vi "Move_Omni_Wheels_Servo.vi"(10 "Spin or not to spin":bool, 11 "Oculus Data":T2={"head"={"orientation"={"roll"=1.6327005330047937, "pitch"=-89.08559793078238, "yaw"=-40.95061142092874}, "position"={"x"=1.207441, "y"=0.483058, "z"=-0.742013}}, "hands"={"left"={"position"={"x"=inf, "y"=inf, "z"=-inf}, "orientation"={"roll"=-51.475846117481964, "pitch"=106.93248840397386, "yaw"=69.74254276716579}}, "right"={"position"={"x"=inf, "y"=inf, "z"=-inf}, "orientation"={"roll"=49.02272731762935, "pitch"=105.46319543414037, "yaw"=-123.9602784132463}}}, "buttons"={"a"=FALSE, "b"=FALSE, "x"=FALSE, "y"=FALSE, "menu"=FALSE, "leftTrig"=1e-06, "rightTrig"=1e-06, "leftGrip"=1e-06, "rightGrip"=1e-06, "left_jstick"={"x"=-0.002561, "y"=0.007201, "button"=FALSE}, "right_jstick"={"x"=0.0, "y"=0.0, "button"=FALSE}}}) -> (3 "2D Picture":picture)   [LabVIEW 2017]
uses:
  <vilib>/myRIO/Instrument Drivers/Onboard IO/PWM/typedefs/PWM Reference.ctl
  <vilib>/myRIO/Common/Instrument Driver Framework/Utilities/typedefs/myRIO Generic Hardware Reference.ctl
  <vilib>/myRIO/Common/Instrument Driver Framework/Utilities/typedefs/Hardware Version Enum.ctl
  <vilib>/myRIO/Common/Instrument Driver Framework/Utilities/typedefs/myRIO v1.0 Reference.ctl
  <vilib>/myRIO/Common/Instrument Driver Framework/Utilities/typedefs/Generic FPGA Reference.ctl
  <vilib>/myRIO/Common/Instrument Driver Framework/myRIO v1.0/PWM/typedefs/PWM Channels Enum.ctl
  <vilib>/myRIO/Instrument Drivers/Onboard IO/PWM/typedefs/PWM Configuration.ctl
  <vilib>/userdefined/High Color/nirio_resource_hc.ctl
  <vilib>/myRIO/Common/Instrument Driver Framework/Utilities/vis/Is FPGA Ref Available.vi
  <vilib>/myRIO/Common/Instrument Driver Framework/myRIO v1.0/PWM/vis/myRIO v1.1 Open PWM.vi
  <vilib>/myRIO/Instrument Drivers/Onboard IO/PWM/vis/Set Duty Cycle and Frequency.vi
  <vilib>/myRIO/Common/Instrument Driver Framework/Utilities/vis/Validate Channels.vi
  <vilib>/myRIO/Common/Instrument Driver Framework/myRIO v1.0/PWM/vis/myRIO v1.0 Reserve PWM.vi
  <vilib>/myRIO/Common/Instrument Driver Framework/myRIO v1.0/PWM/vis/myRIO v1.0 Build MUX Configuration PWM.vi
  <vilib>/myRIO/Common/Instrument Driver Framework/myRIO v1.0/Resource Manager/vis/myRIO v1.0 Reserve Channel List.vi
  <vilib>/myRIO/Common/Instrument Driver Framework/myRIO v1.0/Resource Manager/vis/myRIO v1.0 Create Configuration List.vi
  <vilib>/myRIO/Common/Instrument Driver Framework/myRIO v1.0/Resource Manager/vis/myRIO v1.0 Reserve Channel.vi
  <vilib>/myRIO/Common/Instrument Driver Framework/myRIO v1.0/Resource Manager/vis/myRIO v1.0 Unreserve Channel.vi
  <vilib>/myRIO/Common/Instrument Driver Framework/myRIO v1.0/Resource Manager/vis/myRIO v1.0 Build Mutex Name.vi
  <vilib>/Utility/VariantDataType/GetNumericInfo.vi
  <vilib>/Utility/error.llb/Error Cluster From Error Code.vi
  <vilib>/myRIO/Common/Instrument Driver Framework/myRIO v1.0/myRIO v1.1 Open.vi
  <vilib>/myRIO/Common/Instrument Driver Framework/Utilities/vis/IO Manager.vi
  <vilib>/myRIO/Common/Instrument Driver Framework/Utilities/vis/Configuration Manager.vi
  <vilib>/myRIO/Common/Instrument Driver Framework/myRIO v1.0/Resource Manager/vis/myRIO v1.0 Configure IO.vi
  <vilib>/myRIO/Common/Instrument Driver Framework/myRIO v1.0/myRIO v1.0 Close.vi
  <vilib>/myRIO/Common/Instrument Driver Framework/myRIO v1.0/PWM/vis/myRIO v1.0 Write PWM.vi
  <vilib>/express/express arith-compare/Formula/XNode/ExpressFormulaBlockNode.xnode
  <vilib>/myRIO/Express VI/Onboard IO/PWM/PWM Express VI.xnode
  <vilib>/myRIO/Instrument Drivers/Onboard IO/PWM/vis/myRIO PWM Open.xnode
  <vilib>/myRIO/Instrument Drivers/Onboard IO/PWM/PWM.lvlib
panel:
  in  "rect":T1={"left"=0, "top"=0, "right"=407, "bottom"=407}
  out "r scaled":dbl=1e-06
  in  "Arrow Size":dbl=15.0 format="%#_13g"
  in  "Rotation Radius":dbl=50.0 format="%#_13g"
  out "SuMM":dbl(slide)=2.168404344971009e-18 scale=-3.0..3.0
  out "M3 Slider":dbl(slide)=-0.004955748932651739 scale=-1.0..1.0
  out "M2 Slider":dbl(slide)=0.007516748932651743 scale=-1.0..1.0
  out "M1 Slider":dbl(slide)=-0.002561000000000002 scale=-1.0..1.0
  out "Duty 3":dbl=0.075
  out "Duty 2":dbl=0.075
  out "Duty 1":dbl=0.075
  out "buttons.rightGrip":dbl=1e-06
  out "buttons.leftGrip":dbl=1e-06
  out "RightJoyStick X":dbl(slide) scale=-1.0..1.0
  out "X":dbl=-0.002561
  out "M 3":dbl=-0.004955748932651739
  out "M 2":dbl=0.007516748932651743
  out "M 1":dbl=-0.002561000000000002
  out "Y":dbl=0.007201
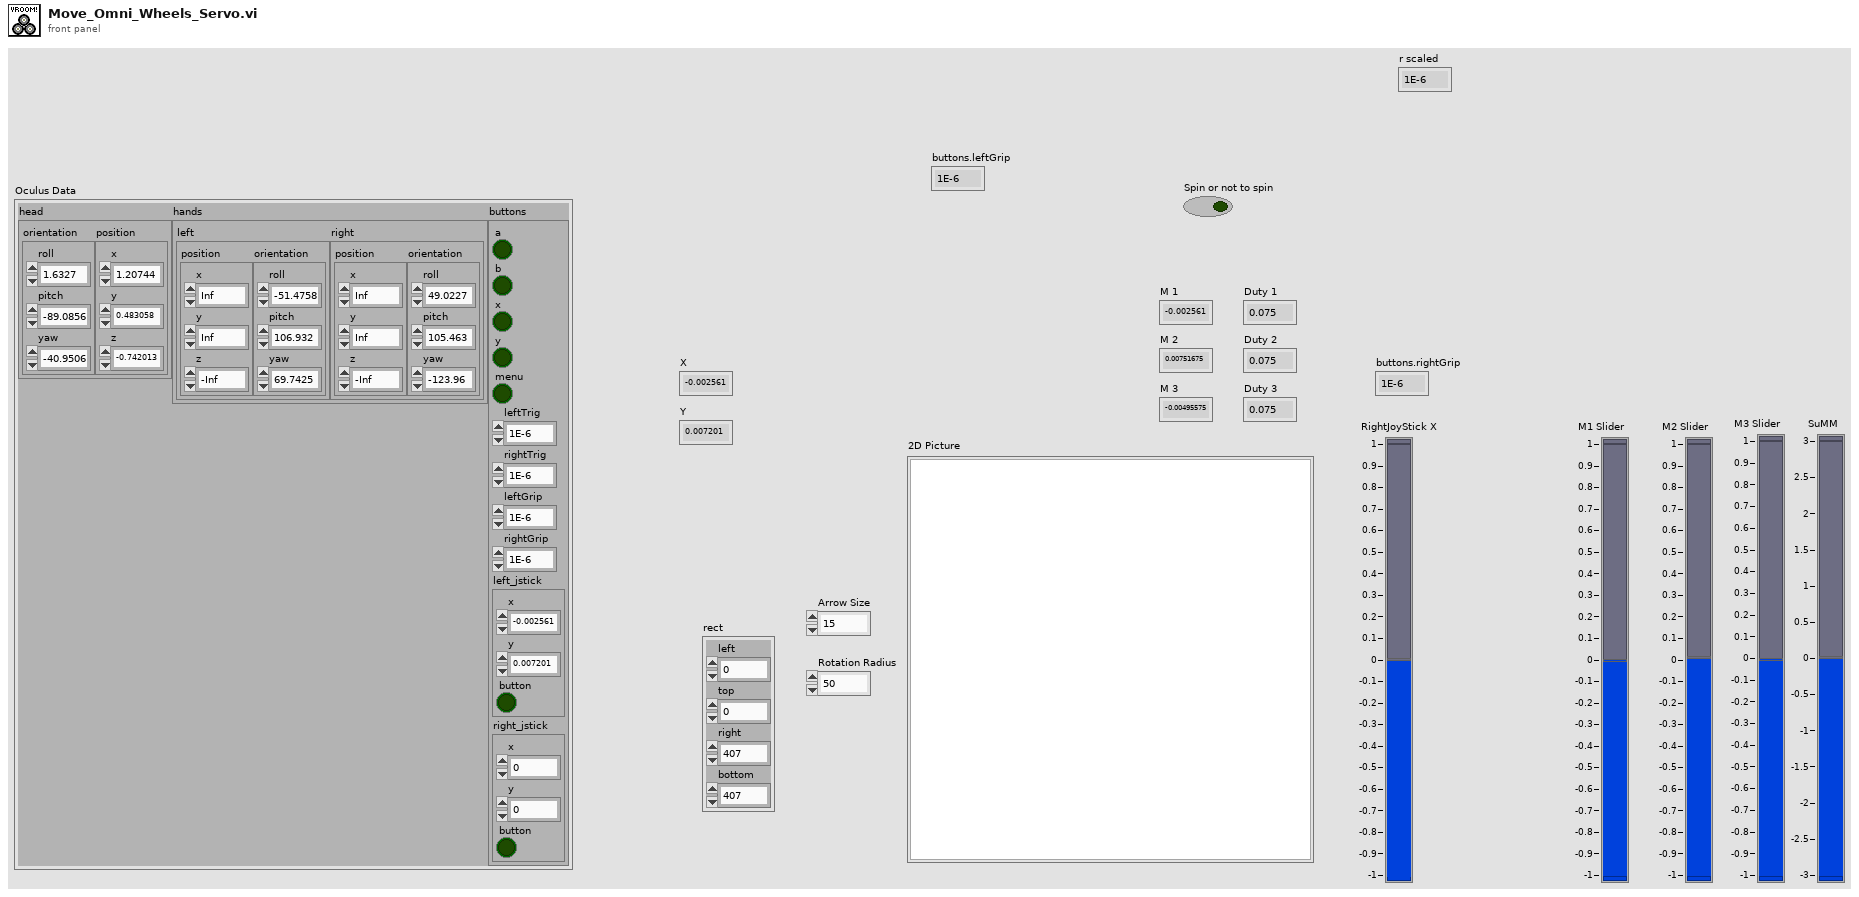
[diagram p1: front panel]
types:
  T1 = cluster{"left":i16, "top":i16, "right":i16, "bottom":i16}
  T2 = cluster{"head":cluster{"orientation":cluster{"roll":dbl, "pitch":dbl, "yaw":dbl}, "position":cluster{"x":dbl, "y":dbl, "z":dbl}}, "hands":cluster{"left":cluster{"position":cluster{"x":dbl, "y":dbl, "z":dbl}, "orientation":cluster{"roll":dbl, "pitch":dbl, "yaw":dbl}}, "right":cluster{"position":cluster{"x":dbl, "y":dbl, "z":dbl}, "orientation":cluster{"roll":dbl, "pitch":dbl, "yaw":dbl}}}, "buttons":cluster{"a":bool, "b":bool, "x":bool, "y":bool, "menu":bool, "leftTrig":dbl, "rightTrig":dbl, "leftGrip":dbl, "rightGrip":dbl, "left_jstick":cluster{"x":dbl, "y":dbl, "button":bool}, "right_jstick":cluster{"x":dbl, "y":dbl, "button":bool}}}
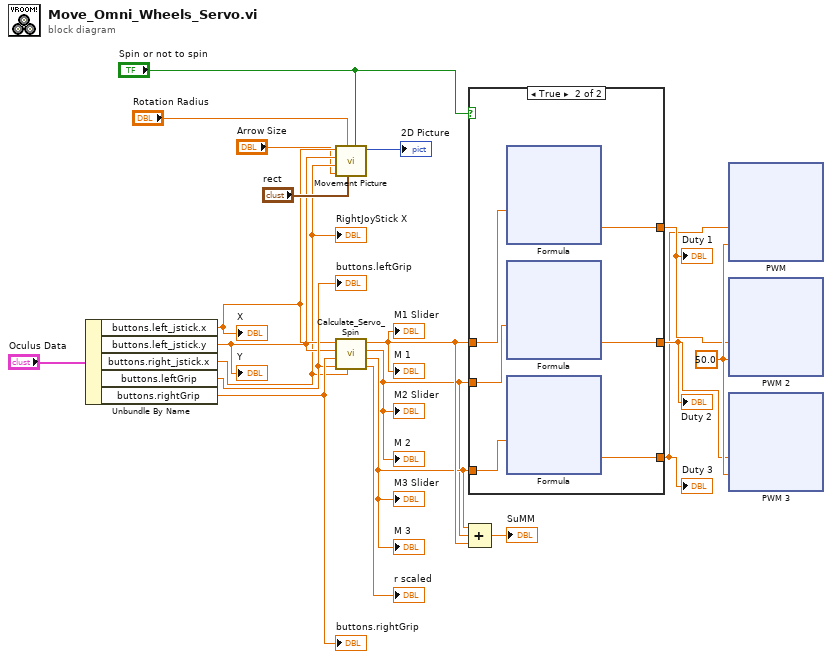
[diagram p0: block diagram]
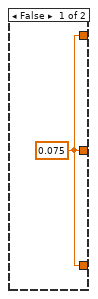
[diagram p2: hidden frame]
diagram:
  w18 = 50.0 ("y")
  n1 = Unbundle By Name("Oculus Data") -> ("buttons.left_jstick.x"=w7:dbl, "buttons.left_jstick.y"=w6:dbl, "buttons.right_jstick.x"=w5:dbl, "buttons.leftGrip"=w16:dbl, "buttons.rightGrip"=w17:dbl)
  "Y" <- w6
  "X" <- w7
  "RightJoyStick X" <- w5
  "buttons.leftGrip" <- w16
  "buttons.rightGrip" <- w17
  n2 = call "Movement Picture.vi"("Spin or not to spin\n(add pause sign in corner if not spinning)"="Spin or not to spin", "rect"="rect", "Rotation Radius"="Rotation Radius", "Arrow Size"="Arrow Size", "RightJoyStick X"=w5, "Y"=w6, "X"=w7) -> ("2D Picture"=→"2D Picture":picture)  [unwired: 4 in]
  n3 = call "Calculate_Servo_Spin.vi"("RightJoyStick X"=w5, "buttons.leftGrip"=w16, "buttons.rightGrip"=w17, "y"=w6, "x"=w7) -> ("r scaled"=→"r scaled":dbl, "M3"=w13:dbl, "M2"=w12:dbl, "M1"=w14:dbl)  [unwired: 3 in]
  "M 1" <- w14
  "M 2" <- w12
  "M 3" <- w13
  "M1 Slider" <- w14
  "M2 Slider" <- w12
  "M3 Slider" <- w13
  n4 = case shown="True" "Spin or not to spin" {
    tunnel: [w21 w27] -> w3
    tunnel: [w21 w26] -> w1
    tunnel: [w21 w25] -> w2
    tunnel: w13 -> [_ w24]
    tunnel: w12 -> [_ w23]
    tunnel: w14 -> [_ w22]
    frame False {
      w21 = 0.075
    }
    frame True {
      n5 = xnode "Formula"("X1"=w22) -> ("Result"=w27:dbl)  [unwired: 1 in, 1 out]
      n6 = xnode "Formula"("X1"=w23) -> ("Result"=w25:dbl)  [unwired: 1 in, 1 out]
      n7 = xnode "Formula"("X1"=w24) -> ("Result"=w26:dbl)  [unwired: 1 in, 1 out]
    }
  }
  "Duty 1" <- w3
  "Duty 2" <- w2
  "Duty 3" <- w1
  n8 = Compound Arithmetic op=ADD(w13, w12, w14) -> (→"SuMM":dbl)
  n9 = xnode "PWM"("Duty Cycle"=w1, "Frequency [Hz]"=w18) -> ()  [unwired: 1 in, 1 out]
  n10 = xnode "PWM 2"("Duty Cycle"=w3, "Frequency [Hz]"=w18) -> ()  [unwired: 1 in, 1 out]
  n11 = xnode "PWM 3"("Duty Cycle"=w2, "Frequency [Hz]"=w18) -> ()  [unwired: 1 in, 1 out]
